vi "Test Timed Functions.vi"() -> ()   [LabVIEW 2017]
panel:
  out "True/False":bool
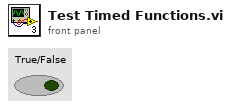
[diagram p1: front panel]
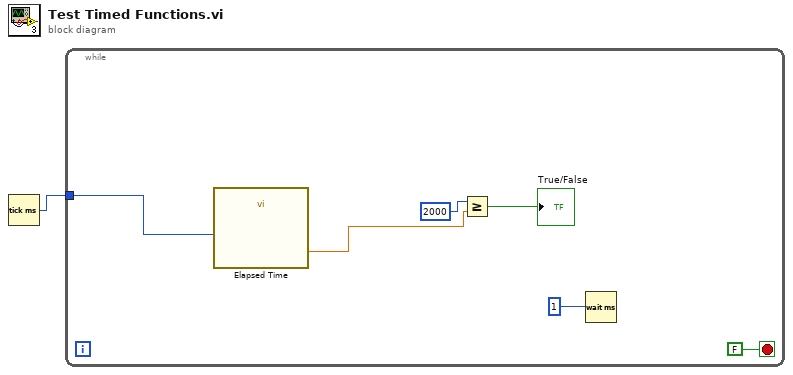
[diagram p0: block diagram]
diagram:
  n1 = Tick Count (ms)() -> (millisecond timer value=w1:u32)
  n2 = while {
    tunnel: w1 -> [w2]
    stop <- FALSE stop-if-true
    n3 = call "Elapsed Time.vi"("Start Time"=w2) -> ("Elapsed Time"=w3:dbl)  [unwired: 10 in]
    n4 = Greater Or Equal?(x=u32 2000 ("y"), y=w3) -> (x >= y?=→"True/False":bool)
    n5 = Wait (ms)(milliseconds to wait=u32 1 ("millisecond timer value")) -> ()  [unwired: 1 out]
  }
